vi "New Interface Error.vi"(7 "error source vi name":string, 11 "error":T1) -> (1 "new offset":i32, 3 "error out":errorcluster)   [LabVIEW 2021, in "DSF Core.lvlib" / "Interface.lvclass"]
uses:
  Interface.lvclass
  Errors.ctl
  <vilib>/NI/Memory Manager/VIs/New Error Cluster (512B).vi
  <vilib>/NI/Memory Manager/Static Errors.lvlib
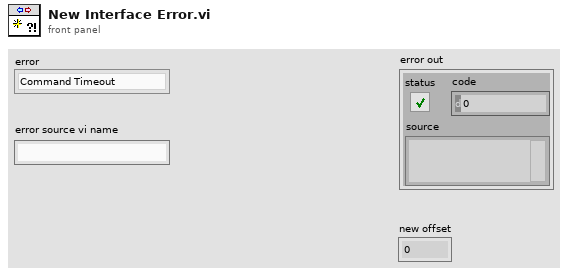
[diagram p1: front panel]
types:
  T1 = typedef "DSF Core.lvlib/Interface.lvclass/Errors.ctl" = enum16{"Command Timeout", "Response Timeout", "Error Timeout", "Invalid Response", "Invalid Response Parameters"}
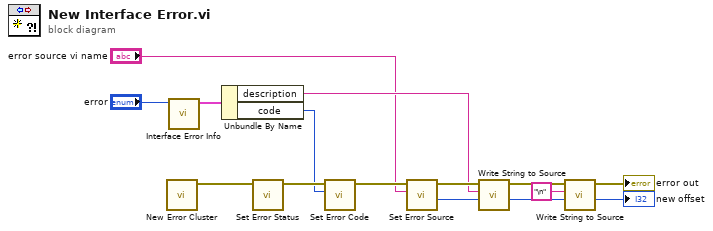
[diagram p0: block diagram]
diagram:
  n1 = call-poly <vilib>:"New Error Cluster.vi"() -> ("error out"=w14:errorcluster)  [unwired: 10 in, 1 out]
  n2 = call "Interface Error Info.vi"("error"="error") -> ("error info"=w12:cluster{"code":i32, "description":string})  [unwired: 10 in]
  n3 = Unbundle By Name(w12) -> ("description"=w7:string, "code"=w11:i32)
  n4 = call <vilib>:"Set Error Status.vi"("error in"=w14) -> ("error out"=w13:errorcluster)  [unwired: 10 in]
  n5 = call <vilib>:"Set Error Code.vi"("code"=w11, "error in"=w13) -> ("error out"=w10:errorcluster)  [unwired: 9 in]
  n6 = call <vilib>:"Set Error Source.vi"("vi name"="error source vi name", "error in"=w10) -> ("initial offset"=w8:i32, "error out"=w9:errorcluster)  [unwired: 8 in]
  n7 = call <vilib>:"Write String to Source.vi"("offset"=w8, "string"=w7, "error in"=w9) -> ("new offset"=w4:i32, "error out"=w6:errorcluster)  [unwired: 7 in]
  n8 = call <vilib>:"Write String to Source.vi"("offset"=w4, "string"="\n", "error in"=w6) -> ("new offset"=→"new offset":i32, "error out"=→"error out":errorcluster)  [unwired: 7 in]
